vi "LabVIEW 2011 - Image Display.vi"() -> ()   [LabVIEW 2017]
panel:
  in  "Close":bool
  out "new picture":picture
  # "Marvin Tester V 1.0.\nDeveloped by Redler Technologies.\nAll rights reserved."
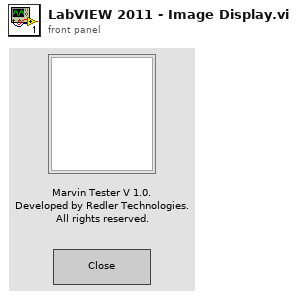
[diagram p1: front panel]
types:
  T1 = typedef "imagedata.ctl" = cluster{"image type":i32, "image depth":i32, "image":u8[], "mask":u8[], "colors":u32[], "Rectangle":cluster{"left":i16, "top":i16, "right":i16, "bottom":i16}}
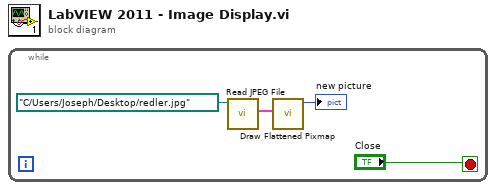
[diagram p0: block diagram]
diagram:
  n1 = while {
    stop <- "Close" stop-if-true
    n2 = call <vilib>:"Read JPEG File.vi"("path to JPEG file"=path "C:/Users/Joseph/Desktop/redler.jpg") -> ("image data"=w4:T1)  [unwired: 8 in, 2 out]
    n3 = call <vilib>:"Draw Flattened Pixmap.vi"("image data"=w4) -> ("new picture"=→"new picture":picture)  [unwired: 8 in]
  }
